vi "ATMonochromator_logEvent_monochromatorConnected.vi"(8 "error in (no error)":errorcluster, 11 "logevent_monochromatorConnected_Ctl":T1) -> (0 "error out":errorcluster, 2 "function return":i32, 3 "logevent_monochromatorConnected_Ctl out":T1)   [LabVIEW 2016, in "SALLV_ATMonochromator.lvlib"]
doc: "int ATMonochromator_shm_logEvent_monochromatorConnectedLV(ATMonochromator_logevent_monochromatorConnectedLV *logevent_monochromatorConnected_Ctl );"
uses:
  SALLV_ATMonochromator.lvlib
  DataTypes/logevent_monochromatorConnected.ctl
  SALLV_ATMonochromator.so
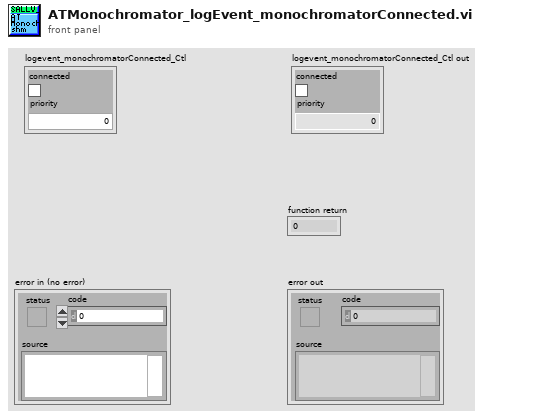
[diagram p1: front panel]
types:
  T1 = typedef "SALLV_ATMonochromator.lvlib/logevent_monochromatorConnected.ctl" = cluster{"connected":bool, "priority":i32}
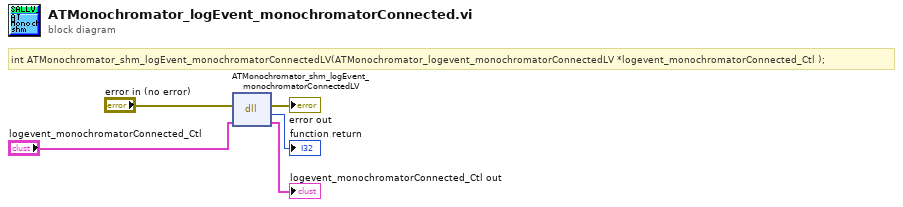
[diagram p0: block diagram]
diagram:
  # "int ATMonochromator_shm_logEvent_monochromatorConnectedLV(ATMonochromator_logevent_monochromatorConnectedLV *logevent_monochromatorConnected_Ctl );"
  n1 = dll-call lib="home/harini/tcs/SALLV_ATMonochromator/SALLV_ATMonochromator.*" fn="ATMonochromator_shm_logEvent_monochromatorConnectedLV"(error in="error in (no error)", "logevent_monochromatorConnected_Ctl"="logevent_monochromatorConnected_Ctl") -> (error out=→"error out":errorcluster, →"function return":i32, "logevent_monochromatorConnected_Ctl"=→"logevent_monochromatorConnected_Ctl out":T1)  [unwired: 2 in, 1 out]
